vi "StackingSensorConvert.vi"() -> (4 "Pos5":u32, 6 "Pos4":u32, 8 "Pos3":u32, 10 "Pos2":u32, 15 "Pos1":u32)   [LabVIEW 2014]
uses:
  Global Variables/Refnum Names.vi
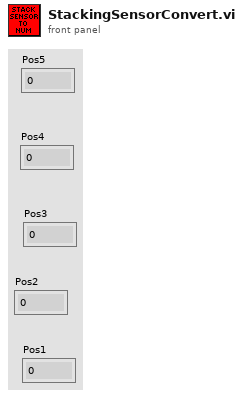
[diagram p1: front panel]
types:
  T1 = typedef "WPI_DigitalInputDevRef.ctl" = cluster{"DevStatus":errorcluster, "DIO Channel":T2, "Controller":T3}
  T2 = typedef "FPGA_DIOChannel.ctl" = enum8{"DIO 0", "DIO 1", "DIO 2", "DIO 3", "DIO 4", "DIO 5", "DIO 6", "DIO 7", "DIO 8", "DIO 9", "DIO MXP 0", "DIO MXP 1", "DIO MXP 2", "DIO MXP 3", "DIO MXP 4", "DIO MXP 5", "DIO MXP 6", "DIO MXP 7", "DIO MXP 8", "DIO MXP 9", "DIO MXP 10", "DIO MXP 11", "DIO MXP 12", "DIO MXP 13", "DIO MXP 14", "DIO MXP 15", "Invalid"}
  T3 = typedef "FPGA_TypedefDigitalModule.ctl" = enum16{"Controller 1"}
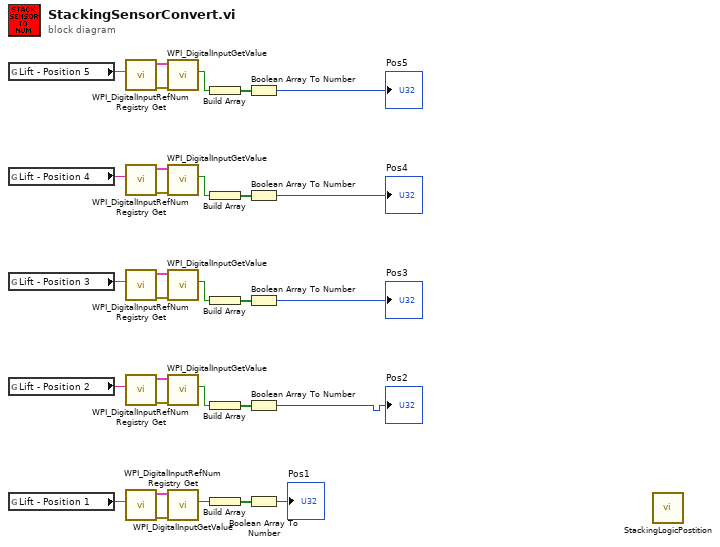
[diagram p0: block diagram]
diagram:
  n1 = global read "Refnum Names.vi" "Lift - Position 5"() -> (w26:string)
  n2 = global read "Refnum Names.vi" "Lift - Position 4"() -> (w27:string)
  n3 = global read "Refnum Names.vi" "Lift - Position 3"() -> (w28:string)
  n4 = global read "Refnum Names.vi" "Lift - Position 2"() -> (w29:string)
  n5 = global read "Refnum Names.vi" "Lift - Position 1"() -> (w30:string)
  n6 = call <vilib>:"WPI_DigitalInputRefNum Registry Get.vi"("refnum name"=w26) -> ("error out"=w16:errorcluster, "DigitalInputDevRef"=w17:T1)  [unwired: 9 in]
  n7 = call <vilib>:"WPI_DigitalInputRefNum Registry Get.vi"("refnum name"=w27) -> ("error out"=w21:errorcluster, "DigitalInputDevRef"=w22:T1)  [unwired: 9 in]
  n8 = call <vilib>:"WPI_DigitalInputRefNum Registry Get.vi"("refnum name"=w28) -> ("error out"=w18:errorcluster, "DigitalInputDevRef"=w23:T1)  [unwired: 9 in]
  n9 = call <vilib>:"WPI_DigitalInputRefNum Registry Get.vi"("refnum name"=w29) -> ("error out"=w19:errorcluster, "DigitalInputDevRef"=w24:T1)  [unwired: 9 in]
  n10 = call <vilib>:"WPI_DigitalInputRefNum Registry Get.vi"("refnum name"=w30) -> ("error out"=w20:errorcluster, "DigitalInputDevRef"=w25:T1)  [unwired: 9 in]
  n11 = call <vilib>:"WPI_DigitalInputGetValue.vi"("error in (no error)"=w16, "DigitalInputDevRef"=w17) -> ("Value"=w4:bool)  [unwired: 7 in, 2 out]
  n12 = call <vilib>:"WPI_DigitalInputGetValue.vi"("error in (no error)"=w21, "DigitalInputDevRef"=w22) -> ("Value"=w9:bool)  [unwired: 7 in, 2 out]
  n13 = call <vilib>:"WPI_DigitalInputGetValue.vi"("error in (no error)"=w18, "DigitalInputDevRef"=w23) -> ("Value"=w8:bool)  [unwired: 7 in, 2 out]
  n14 = call <vilib>:"WPI_DigitalInputGetValue.vi"("error in (no error)"=w19, "DigitalInputDevRef"=w24) -> ("Value"=w7:bool)  [unwired: 7 in, 2 out]
  n15 = call <vilib>:"WPI_DigitalInputGetValue.vi"("error in (no error)"=w20, "DigitalInputDevRef"=w25) -> ("Value"=w15:bool)  [unwired: 7 in, 2 out]
  n16 = Build Array(w4) -> (w10:bool[])
  n17 = Build Array(w9) -> (w11:bool[])
  n18 = Build Array(w8) -> (w12:bool[])
  n19 = Build Array(w7) -> (w13:bool[])
  n20 = Build Array(w15) -> (w14:bool[])
  n21 = Boolean Array To Number(Boolean array=w10) -> (number=→"Pos5":u32)
  n22 = Boolean Array To Number(Boolean array=w11) -> (number=→"Pos4":u32)
  n23 = Boolean Array To Number(Boolean array=w12) -> (number=→"Pos3":u32)
  n24 = Boolean Array To Number(Boolean array=w13) -> (number=→"Pos2":u32)
  n25 = Boolean Array To Number(Boolean array=w14) -> (number=→"Pos1":u32)
  n26 = call "StackingLogicPostition.vi"() -> ()  [unwired: 12 in]
